vi "Set SG Path.vi"(0 "Path in":refnum<class "SA 8GHz Path.lvclass">, 5 "Cal point in":T1, 11 "error in":errorcluster) -> (4 "Path out":refnum<class "SA 8GHz Path.lvclass">, 6 "Cal point out":T1, 8 "Source Gain":dbl, 10 "Digital Gain":dbl, 15 "error out":errorcluster)   [LabVIEW 2023, in "RFFixtureCharact.RMM.lvlib" / "SA 8GHz Path.lvclass"]
uses:
  Public/Base Classes/Scalar/Scalar Path/Type Definitions/Cal Point.ctl
  Public/Base Classes/Scalar/SA Abstract Path/SA Abstract Path.lvclass/SA Abstract Path.ctl
  Public/Base Classes/Scalar/SA Abstract Path/Properties/Read Cal Tone Pin.vi
  SA 8GHz Path.lvclass
  SA 8GHz Path.lvclass/SA 8GHz Path.ctl
  Public/Base Classes/Scalar/SA Path/SA Path.lvclass
  Public/Base Classes/Scalar/Scalar Path/Scalar Path.lvclass
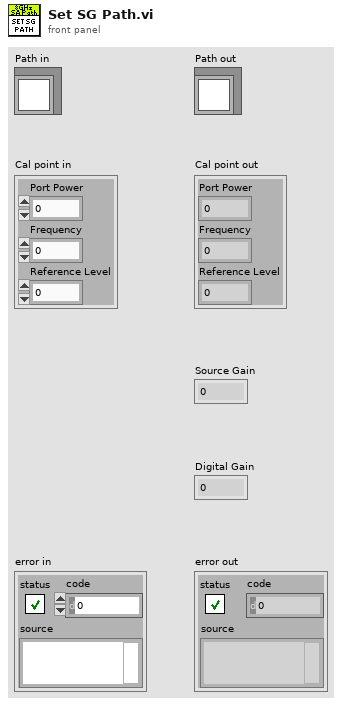
[diagram p1: front panel]
types:
  T1 = typedef "RFFixtureCharact.Public.lvlib/Scalar Path.lvclass/Cal Point.ctl" = cluster{"Port Power":dbl, "Frequency":dbl, "Reference Level":dbl}
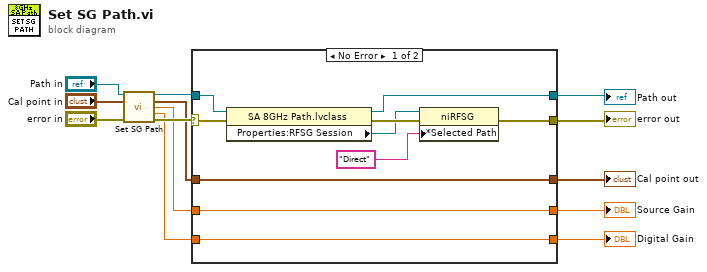
[diagram p0: block diagram]
diagram:
  n1 = call-parent "Set SG Path.vi"("Path in"="Path in", "Cal point in"="Cal point in", "error in"="error in") -> ("Path out"=w4:refnum<class "SA 8GHz Path.lvclass">, "Cal point out"=w2:T1, "Source Gain"=w3:dbl, "Digital Gain"=w1:dbl, "error out"=w9:errorcluster)  [unwired: 8 in]
  n2 = case shown="No Error" w9 {
    selector: w9 -> [w23 w28]
    tunnel: w4 -> [w22 w27]
    tunnel: [w19 w27] -> w5
    tunnel: [w18 w28] -> w10
    tunnel: [w16 w26] -> w6
    tunnel: w2 -> [w16 w26]
    tunnel: [w15 w25] -> w7
    tunnel: w3 -> [w15 w25]
    tunnel: [w14 w24] -> w8
    tunnel: w1 -> [w14 w24]
    frame No Error {
      n3 = property class="SA 8GHz Path.lvclass"(reference=w22, error in=w23) -> (reference out=w19:refnum<class "SA 8GHz Path.lvclass">, error out=w21:errorcluster, "Properties:RFSG Session"=w20:refnum<k15>)
      n4 = property class="niRFSG"(reference=w20, error in=w21, "*Selected Path"="Direct" ("Private:Device Specific:Vector Signal Transceiver:Signal Path:Selected Path")) -> (error out=w18:errorcluster)  [unwired: 1 out]
    }
    frame Error {
    }
  }
  "error out" <- w10
  "Source Gain" <- w7
  "Cal point out" <- w6
  "Digital Gain" <- w8
  "Path out" <- w5
